vi "TimeInterpBoolean_GetSample.vi"(9 "TimeStamp":dbl, 11 "TimeInterpBoolean":T1) -> (1 "IsPresent":bool, 3 "OutputBoolean":bool)   [LabVIEW 2019, in "Trajectory_Library.lvlib"]
doc: "Sample the buffer at the given time.\n\nThis retuns the value sample at or before the requested time. (boolean values can't be interpolated.)\n\nInputs:\n - TimeInterpBoolean -- Input data cluster\n - TimeStamp -- Time at which to sample (seconds)\n\nOutputs\n - OutputBoolean -- Sampled boolean. This is an exact value if there is a sample in the buffer at this time. Otherwise it is the next previous sample.\n - IsPresent -- Returns TRUE if the buffer contains data as far back as TimeStamp."
uses:
  Trajectory_Library.lvlib
  TypeDef/TIME_INTERPOLATABLE_BOOLEAN.ctl
  <vilib>/gmath/NI_Gmath.lvlib
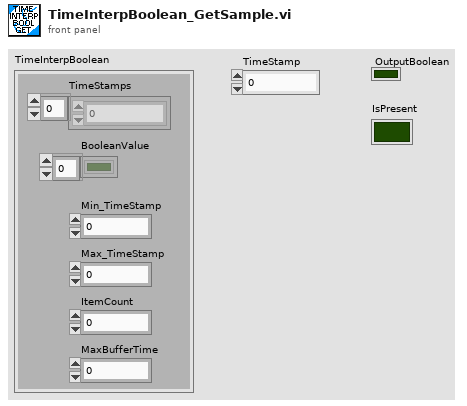
[diagram p1: front panel]
types:
  T1 = typedef "Trajectory_Library.lvlib/TIME_INTERPOLATABLE_BOOLEAN.ctl" = cluster{"TimeStamps":dbl[], "BooleanValue":bool[], "Min_TimeStamp":dbl, "Max_TimeStamp":dbl, "ItemCount":i32, "MaxBufferTime":dbl}
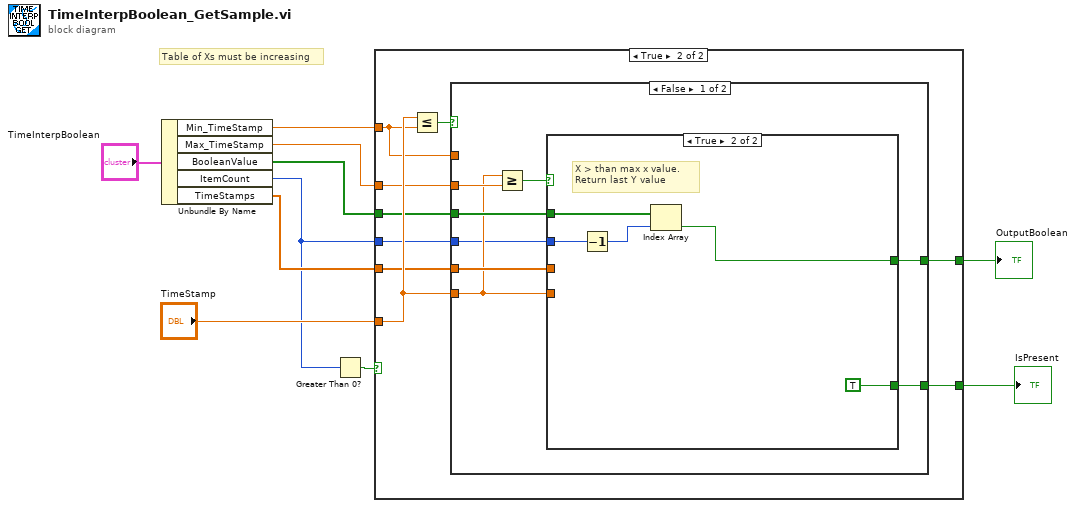
[diagram p0: block diagram]
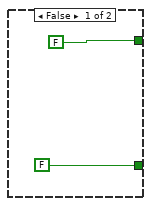
[diagram p2: hidden frame]
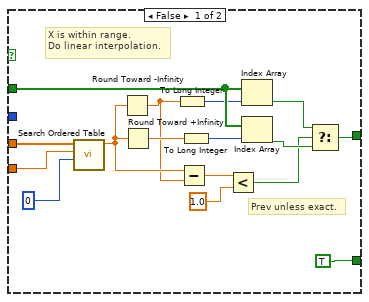
[diagram p3: hidden frame]
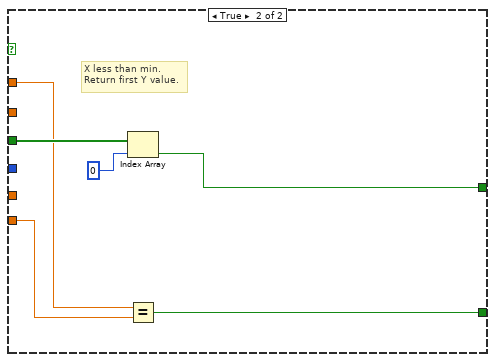
[diagram p4: hidden frame]
diagram:
  # "Table of Xs must be increasing"
  n1 = Unbundle By Name("TimeInterpBoolean") -> ("Min_TimeStamp"=w7:dbl, "Max_TimeStamp"=w6:dbl, "BooleanValue"=w4:bool[], "ItemCount"=w2:i32, "TimeStamps"=w5:dbl[])
  n2 = Greater Than 0?(x=w2) -> (x > 0?=w3:bool)
  n3 = case shown="True" w3 {
    tunnel: "TimeStamp" -> [_ w20]
    tunnel: [FALSE w19] -> w9
    tunnel: w7 -> [_ w14]
    tunnel: w6 -> [_ w18]
    tunnel: w2 -> [_ w17]
    tunnel: w5 -> [_ w16]
    tunnel: w4 -> [_ w15]
    tunnel: [FALSE w13] -> w1
    frame False {
    }
    frame True {
      n4 = Less Or Equal?(x=w20, y=w14) -> (x <= y?=w21:bool)
      n5 = case shown="False" w21 {
        tunnel: w15 -> [w27 w56]
        tunnel: [w26 w54] -> w19
        tunnel: w20 -> [w24 w52]
        tunnel: w18 -> [w29 _]
        tunnel: w16 -> [w25 _]
        tunnel: w17 -> [w23 _]
        tunnel: w14 -> [_ w53]
        tunnel: [w22 w51] -> w13
        frame False {
          n6 = Greater Or Equal?(x=w24, y=w29) -> (x >= y?=w28:bool)
          n7 = case shown="True" w28 {
            tunnel: w27 -> [w42 w50]
            tunnel: [w36 w49] -> w26
            tunnel: w25 -> [w44 _]
            tunnel: w24 -> [w43 _]
            tunnel: w23 -> [_ w48]
            tunnel: [TRUE TRUE] -> w22
            frame False {
              # "Prev unless exact."
              # "X is within range.  \nDo linear interpolation."
              n8 = call <vilib>:"Search Ordered Table.vi"("starting index"=0, "x value"=w43, "ordered x array"=w44) -> ("fractional index"=w38:dbl)  [unwired: 8 in]
              n9 = Round Toward -Infinity(1:w38) -> (0:w37:dbl)
              n10 = Round Toward +Infinity(x=w38) -> (ceil(x): smallest int >= x=w39:dbl)
              n11 = To Long Integer(number=w37) -> (32bit integer=w41:i32)
              n12 = Subtract(x=w38, y=w37) -> (x-y=w33:dbl)
              n13 = To Long Integer(number=w39) -> (32bit integer=w40:i32)
              n14 = Less?(x=w33, y=1.0) -> (x < y?=w31:bool)
              n15 = Index Array(array=w42, index=w41) -> (element=w35:bool)
              n16 = Index Array(array=w42, index=w40) -> (element=w34:bool)
              n17 = Select(t=w35, s=w31, f=w34) -> (s? t:f=w36:bool)
            }
            frame True {
              # "X > than max x value.   \nReturn last Y value"
              n18 = Decrement(x=w48) -> (x-1=w47:i32)
              n19 = Index Array(array=w50, index=w47) -> (element=w49:bool)
            }
          }
        }
        frame True {
          # "X less than min.   \nReturn first Y value."
          n20 = Index Array(array=w56, index=0) -> (element=w54:bool)
          n21 = Equal?(x=w53, y=w52) -> (x = y?=w51:bool)
        }
      }
    }
  }
  "OutputBoolean" <- w9
  "IsPresent" <- w1
